vi "equipoSeleccionado.vi"(8 "error in (no error)":errorcluster, 11 "Calibrador in":refnum<class "Calibrador.lvclass">) -> (0 "error out":errorcluster, 2 "equipoSeleccionado":string, 3 "Calibrador out":refnum<class "Calibrador.lvclass">)   [LabVIEW 2019, in "Calibrador.lvclass"]
uses:
  Calibrador.lvclass
  Calibrador.lvclass/Calibrador.ctl
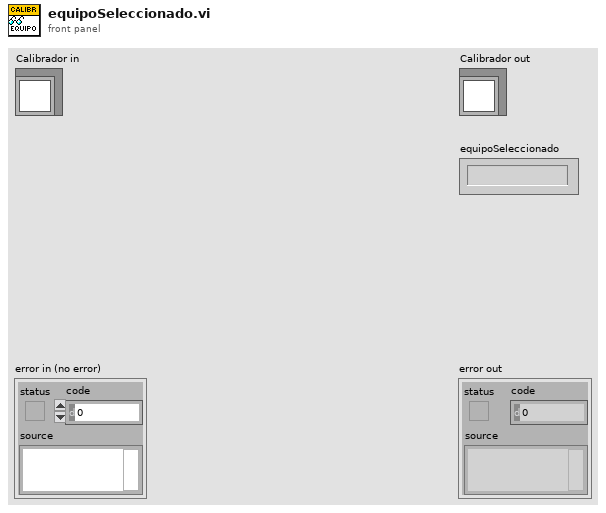
[diagram p1: front panel]
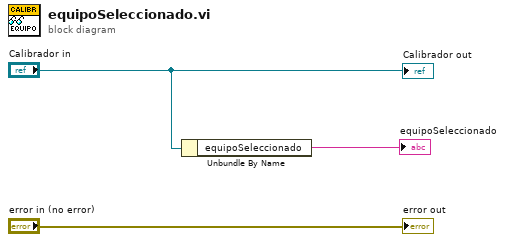
[diagram p0: block diagram]
diagram:
  n1 = Unbundle By Name("Calibrador in") -> ("equipoSeleccionado"=→"equipoSeleccionado":string)
  "error out" <- "error in (no error)"
  "Calibrador out" <- "Calibrador in"
